vi "Get All Environment Variables [Map].vi"(7 "Target (Process)":T1 items=["Process", "User", "Machine"], 8 "Error In":errorcluster) -> (0 "Error Out":errorcluster, 3 "Variables":map{string, string}(c390))   [LabVIEW 2023, in "SLL Environment Variable.lvlib"]
doc: "Retrieve all environment variables and their values from the target environment in a map."
uses:
  SLL Environment Variable.lvlib
  _Typedef/Target Environment Enum.ctl
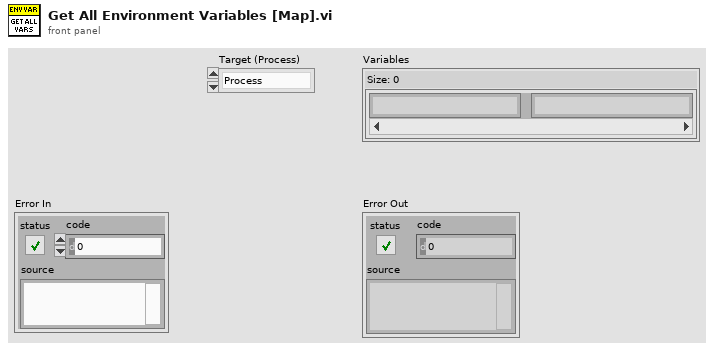
[diagram p1: front panel]
types:
  T1 = typedef "SLL Environment Variable.lvlib/Target Environment Enum.ctl" = i32
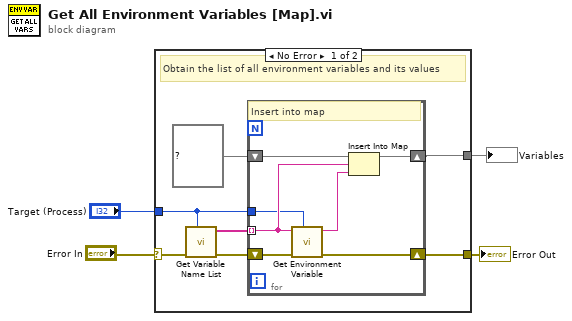
[diagram p0: block diagram]
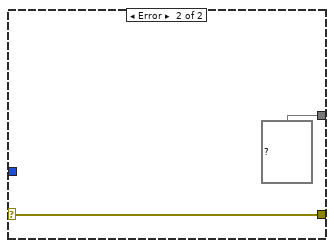
[diagram p2: hidden frame]
diagram:
  n1 = case shown="No Error" "Error In" {
    selector: "Error In" -> [w7 w20]
    tunnel: [w11 w20] -> w4
    tunnel: [w9 map{string, string} {} ("map in")] -> w2
    tunnel: "Target (Process)" -> [w5 _]
    frame No Error {
      # "Obtain the list of all environment variables and its values"
      n2 = call "Get Variable Name List.vi"("Target (Process)"=w5, "Error In"=w7) -> ("Error Out"=w8:errorcluster, "Names[]"=w6:string[])  [unwired: 8 in]
      n3 = for {
        shift-right: [w17] -> w11
        shift-left: w8 -> [w18]
        tunnel: w6 -> [w14] mode=indexing
        shift-right: [w15] -> w9
        shift-left: map{string, string} {} ("map in") -> [w16]
        tunnel: w5 -> [w12]
        # "Insert into map"
        n4 = call "Get Environment Variable.vi"("Target (Process)"=w12, "Error In"=w18, "Name"=w14) -> ("Error Out"=w17:errorcluster, "Value"=w13:string)  [unwired: 7 in]
        n5 = Insert Into Map(map in=w16, key=w14, value=w13) -> (map out=w15:map{string, string})  [unwired: 2 out]
      }
    }
    frame Error {
    }
  }
  "Error Out" <- w4
  "Variables" <- w2
